vi "test_connection_SQUID.vi"(8 "error in (no error)":errorcluster caption="エラー入力（エラーなし）", 11 "VISAリソース名":refnum<visa-resource-name>) -> (0 "error out":errorcluster caption="エラー出力", 2 "connected?":bool, 3 "VISAリソース名（出力）":refnum<visa-resource-name>)   [LabVIEW 2017]
uses:
  <vilib>/Instr/_visa.llb/VISA Configure Serial Port (Instr).vi
panel:
  out "レスポンス":string
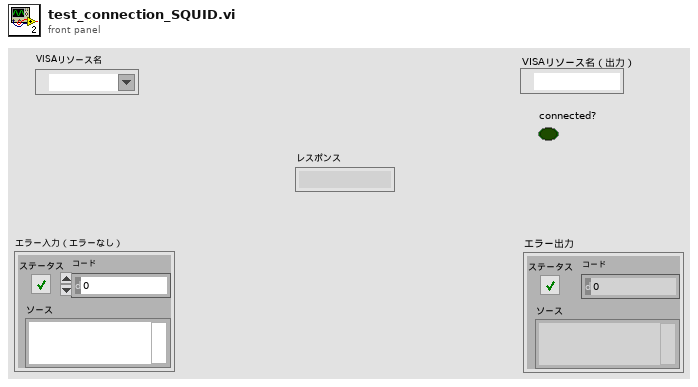
[diagram p1: front panel]
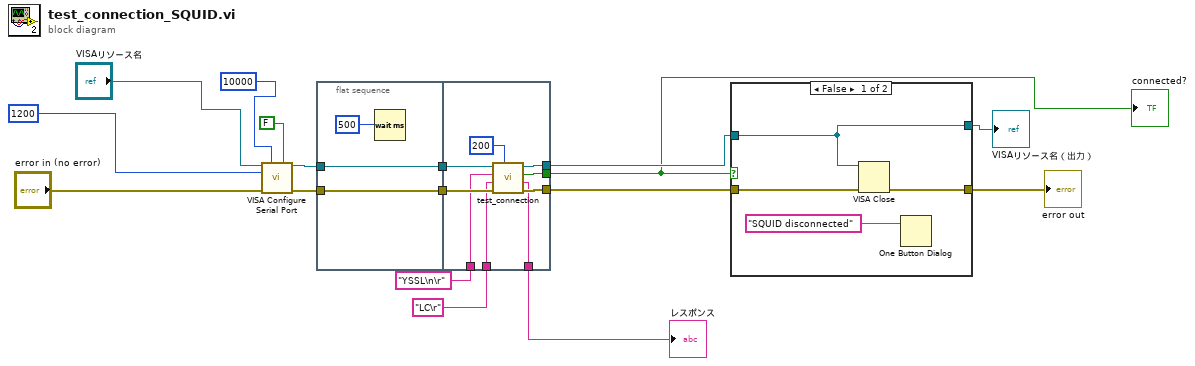
[diagram p0: block diagram]
diagram:
  n1 = call-poly "VISA Configure Serial Port"("VISA resource name"="VISAリソース名", "timeout (10sec)"=10000, "Enable Termination\nChar (T)"=FALSE, "baud rate (9600)"=1200, "error in (no error)"="error in (no error)") -> ("VISA resource name out"=w14:refnum<visa-resource-name>, "error out"=w13:errorcluster)  [unwired: 9 in]
  n2 = flat-sequence {
    tunnel: [w20] -> w8
    tunnel: [w19] -> w7
    tunnel: w14 -> [w20]
    tunnel: w13 -> [w19]
    tunnel: w8 -> [w22]
    tunnel: w7 -> [w28]
    tunnel: "LC\r" ("想定レスポンス") -> [w27]
    tunnel: "YSSL\n\r" ("コマンド") -> [w26]
    tunnel: [w25] -> w4
    tunnel: [w24] -> w2
    tunnel: [w23] -> w3
    tunnel: [w21] -> w1
    frame #0 {
      n3 = Wait (ms)(milliseconds to wait=500) -> ()  [unwired: 1 out]
    }
    frame #1 {
      n4 = call "test_connection.vi"("文字送信間隔 (500 ms)"=200, "error in (no error)"=w28, "想定レスポンス"=w27, "コマンド"=w26, "VISAリソース名"=w22) -> ("error out"=w25:errorcluster, "レスポンス"=w21:string, "一致？"=w24:bool, "VISAリソース名 （出力）"=w23:refnum<visa-resource-name>)  [unwired: 3 in]
    }
  }
  n5 = case shown="FALSE" w2 {
    tunnel: w4 -> [w33 w35]
    tunnel: w3 -> [w30 w34]
    tunnel: [w31 w35] -> w17
    tunnel: [w30 w34] -> w10
    frame False {
      n6 = VISA Close(VISA resource name=w30, error in (no error)=w33) -> (error out=w31:errorcluster)
      n7 = One Button Dialog(message="SQUID disconnected") -> ()  [unwired: 1 in, 1 out]
    }
    frame True {
    }
  }
  "error out" <- w17
  "VISAリソース名（出力）" <- w10
  "connected?" <- w2
  "レスポンス" <- w1
